vi "Load to memory.vi"(0 "LV Doc in":refnum<class "LV Doc.lvclass">, 5 "Path":path, 7 "Batch File Path":path, 11 "error in (no error)":errorcluster) -> (4 "LV Doc out":refnum<class "LV Doc.lvclass">, 6 "Names[]":string[](array[string]), 8 "Child Window Data":T1, 15 "error out":errorcluster)   [LabVIEW 2016, in "LV Doc.lvclass"]
uses:
  LV Doc.lvclass
  Private/Child Window Data.ctl
  LV Doc.lvclass/LV Doc.ctl
  LV MDI.lvclass
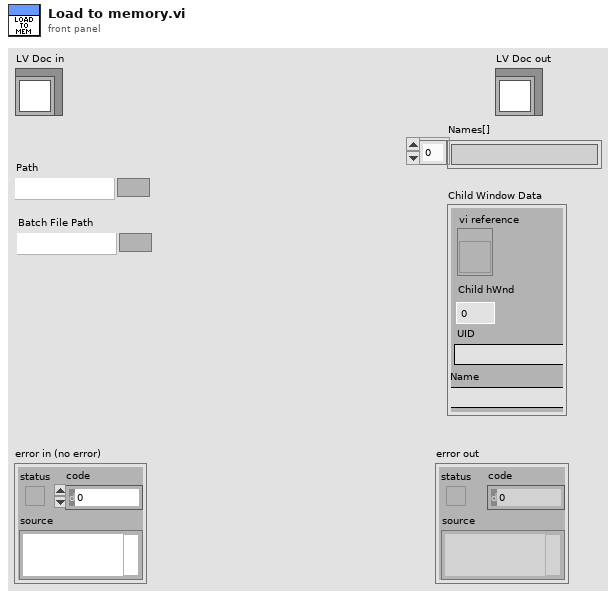
[diagram p1: front panel]
types:
  T1 = typedef "LV MDI.lvclass/Child Window Data.ctl" = cluster{"Child hWnd":u32, "UID":string, "vi reference":refnum<vi>, "Name":string}
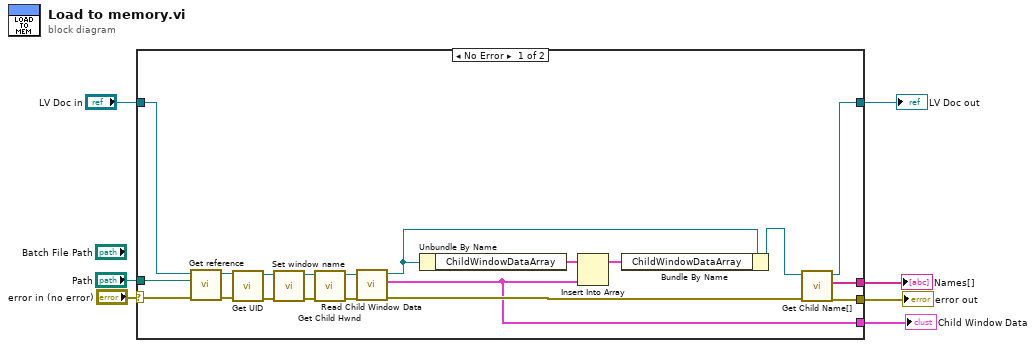
[diagram p0: block diagram]
diagram:
  n1 = case shown="No Error" "error in (no error)" {
    selector: "error in (no error)" -> [w13 w29]
    tunnel: [w12 w29] -> w6
    tunnel: "LV Doc in" -> [w11 w28]
    tunnel: [w10 w28] -> w4
    tunnel: [w14 _] -> w3
    tunnel: "Path" -> [w9 _]
    tunnel: [w8 _] -> w1
    frame No Error {
      n2 = call "Get reference.vi"("Error in"=w13, "Vi Path"=w9, "LV Doc.lvclass"=w11) -> ("Error Out"=w23:errorcluster, "LV Doc.lvclass"=w27:refnum<class "LV Doc.lvclass">)  [unwired: 7 in]
      n3 = call "Get UID.vi"("error in (no error)"=w23, "LV Doc.lvclass"=w27) -> ("error out"=w22:errorcluster, "LV Doc.lvclass"=w26:refnum<class "LV Doc.lvclass">)  [unwired: 8 in]
      n4 = call "Set window name.vi"("error in (no error)"=w22, "LV Doc.lvclass"=w26) -> ("error out"=w21:errorcluster, "LV Doc.lvclass"=w25:refnum<class "LV Doc.lvclass">)  [unwired: 8 in]
      n5 = call "Get Child Hwnd.vi"("Error in"=w21, "LV Doc.lvclass"=w25) -> ("Error Out"=w20:errorcluster, "LV Doc.lvclass"=w24:refnum<class "LV Doc.lvclass">)  [unwired: 8 in]
      n6 = call-dynamic "Read Child Window Data.vi"("error in (no error)"=w20, "LV Doc in"=w24) -> ("error out"=w16:errorcluster, "Child Window Data"=w8:T1, "LV Doc out"=w17:refnum<class "LV Doc.lvclass">)  [unwired: 7 in]
      n7 = Unbundle By Name(w17) -> ("ChildWindowDataArray"=w18:T1[])
      n8 = Insert Into Array(array=w18, new element=w8) -> (w19:T1[])  [unwired: 1 in]
      n9 = Bundle By Name(cluster=w17, "ChildWindowDataArray"=w19) -> (w15:refnum<class "LV Doc.lvclass">)
      n10 = call "Get Child Name[].vi"("error in (no error)"=w16, "LV Doc.lvclass"=w15) -> ("error out"=w12:errorcluster, "Array"=w14:string[], "LV Doc.lvclass"=w10:refnum<class "LV Doc.lvclass">)  [unwired: 7 in]
    }
    frame Error {
    }
  }
  "error out" <- w6
  "LV Doc out" <- w4
  "Names[]" <- w3
  "Child Window Data" <- w1
